vi "Create (Dimensions).vi"(8 "error in (no error)":errorcluster, 10 "Dimensions":i32[](array[numeric]), 11 "U8 array in":u8[](array[numeric])) -> (0 "error out":errorcluster, 3 "Uint8Array out":refnum<class "Uint8Array.lvclass">)   [LabVIEW 2013, in "MDSplus.lvlib" / "Uint8Array.lvclass"]
uses:
  <vilib>/MDSplus/Classes/Data_Class/Array_Class/Uint8Array_Class/Uint8Array.lvclass
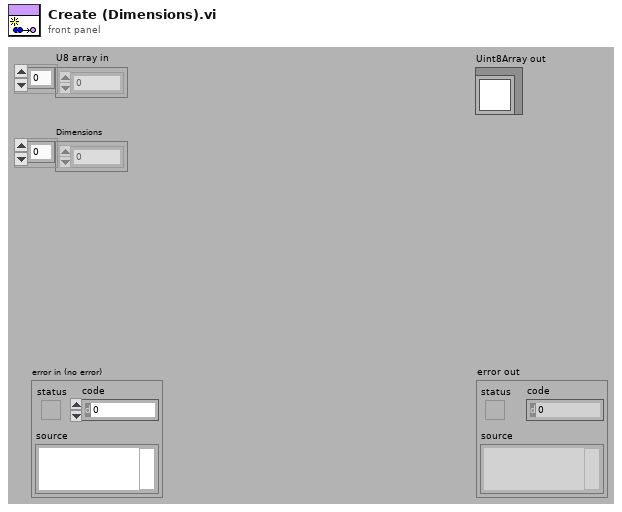
[diagram p1: front panel]
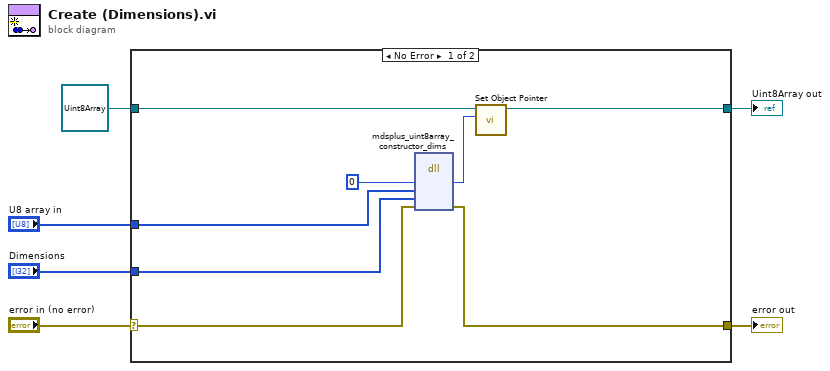
[diagram p0: block diagram]
diagram:
  n1 = case shown="No Error" "error in (no error)" {
    selector: "error in (no error)" -> [w12 w16]
    tunnel: [w7 w16] -> w5
    tunnel: [w10 w15] -> w3
    tunnel: refnum<class "Uint8Array.lvclass"> refnum ("Float32 in") -> [w11 w15]
    tunnel: "U8 array in" -> [w9 _]
    tunnel: "Dimensions" -> [w8 _]
    frame No Error {
      n2 = dll-call lib="MDSobjectsLVShr" fn="mdsplus_uint8array_constructor_dims"("lvUint8ArrayPtrOut"=i64 0 ("lvTreePtr"), "lvUByteArrHdlIn"=w9, "lvIntArrHdlIn"=w8, "error"=w12) -> ("lvUint8ArrayPtrOut"=w13:i64, "error"=w7:errorcluster)  [unwired: 6 in, 2 out]
      n3 = call-dynamic "Set Object Pointer.vi"("Object Pointer"=w13, "Data in"=w11) -> ("Data out"=w10:refnum<class "Uint8Array.lvclass">)  [unwired: 9 in]
    }
    frame Error {
    }
  }
  "error out" <- w5
  "Uint8Array out" <- w3
